vi "Enable.vi"(0 "Interface in":refnum<k20>, 11 "error in":errorcluster) -> (4 "Interface out":refnum<k20>, 15 "error out":errorcluster)   [LabVIEW 2017]
uses:
  InterfaceRef.ctl
  AFE_interface.lvlib
  <vilib>/rvi/interface/nirviReadWriteControl/nirviReadWriteControl.xnode
  NiFpgaLv.dll
  <vilib>/Utility/error.llb/Error Cluster From Error Code.vi
  <vilib>/rvi/interface/Simulation/niFpgaSimulationCallBeginRW.vi
  <vilib>/rvi/errors/niLvFpgaAdjustHostInterfaceError.vi
  <instrlib>/_niInstr/Instruction Framework/v1/Host/Instruction Framework Context/niInstr Instruction Framework Context v1 Host.lvclass
  <instrlib>/_niInstr/Instruction Framework/v1/Host/Instruction Target/niInstr Instruction Target v1 Host.lvclass
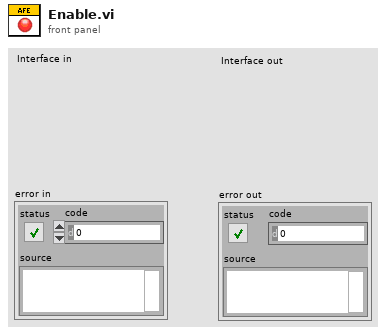
[diagram p1: front panel]
types:
  T1 = typedef "AFE_interface.lvlib/InterfaceRef.ctl" = cluster{"instruction target":refnum<class "niInstr Instruction Target v1 Host.lvclass">, "context":refnum<class "niInstr Instruction Framework Context v1 Host.lvclass">}
  T2 = typedef "AFE_interface.lvlib/InterfaceRef.ctl" = refnum<k20>
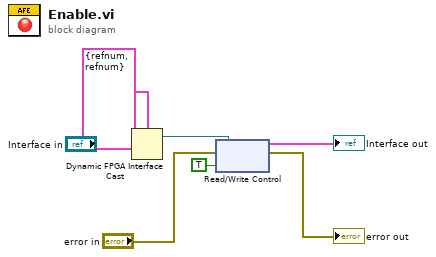
[diagram p0: block diagram]
diagram:
  n1 = Dynamic FPGA Interface Cast(Session In=T1 {"instruction target"=refnum, "context"=refnum} ("Type"), Type="Interface in") -> (Session Out=w5:T2)
  n2 = xnode "Read/Write Control"("FPGA VI Reference In"=w5, "error in"="error in", "enable"=TRUE) -> ("FPGA VI Reference Out"=→"Interface out":T1, "error out"=→"error out":errorcluster)
